vi "log analysis_gps.vi"() -> ()   [LabVIEW 2019] (continued)
system status\tnormal 2 28.000000 0 0\trobot status\t283.924052\t71.154342\t9.753100\t-0.332297\t-2.244729\t149.990746\t0.281000\t0.028000\n\t\n15:33:22.5\tlog_raw\tgps_raw\t#DUALANTENNAHEADINGA,USB3,0,50.5,FINESTEERING,2107,282820.500,02008000,d426,15824;INSUFFICIENT_OBS,NONE,-1.000000000,0.000000000,0.000000000,0.0,0.000000000,0.000000000,\"631T\",14,2,2,2,04,00,20,00*d6a33192\n\tsystem status\tnormal 2 28.000000 0 0\trobot status\t283.808490\t71.236602\t9.749900\t-0.277262\t-2.162787\t150.076452\t0.284000\t0.021000\n\t\n15:33:23.0\tlog_raw\tgps_raw\t#DUALANTENNAHEADINGA,USB3,0,50.5,FINESTEERING,2107,282821.000,02008000,d426,15824;INSUFFICIENT_OBS,NONE,-1.000000000,0.000000000,0.000000000,0.0,0.000000000,0.000000000,\"631T\",16,2,2,2,04,00,20,00*18dc22e3\n\tsystem status\tnormal 2 28.000000 0 0\trobot status\t283.690413\t71.319846\t9.746300\t-0.267508\t-2.122984\t150.127557\t0.314000\t-0.023000\n\t\n15:33:23.5\tlog_raw\tgps_raw\t\tsystem status\tnormal 2 28.000000 0 0\trobot status\t283.569355\t71.402549\t9.742500\t-0.374264\t-1.857958\t150.068560\t0.286000\t0.008000\n\t\n15:33:24.0\tlog_raw\tgps_raw\t#DUALANTENNAHEADINGA,USB3,0,50.0,FINESTEERING,2107,282822.000,02008000,d426,15824;INSUFFICIENT_OBS,NONE,-1.000000000,0.000000000,0.000000000,0.0,0.000000000,0.000000000,\"631T\",16,2,2,2,04,00,20,00*fbcec944\n\tsystem status\tnormal 2 28.000000 0 0\trobot status\t283.449551\t71.484070\t9.737500\t-0.512487\t-1.771439\t150.084314\t0.227000\t0.089000\n\t\n15:33:24.5\tlog_raw\tgps_raw\t#DUALANTENNAHEADINGA,USB3,0,49.0,FINESTEERING,2107,282822.500,02008000,d426,15824;INSUFFICIENT_OBS,NONE,-1.000000000,0.000000000,0.000000000,0.0,0.000000000,0.000000000,\"631T\",15,2,2,2,04,00,20,00*aed41295\n\tsystem status\tnormal 2 28.000000 0 0\trobot status\t283.332205\t71.563886\t9.733200\t-0.549068\t-1.653823\t150.119212\t0.315000\t-0.042000\n\t\n15:33:25.0\tlog_raw\tgps_raw\t#DUALANTENNAHEADINGA,USB3,0,49.0,FINESTEERING,2107,282823.000,02008000,d426,15824;INSUFFICIENT_OBS,NONE,-1.000000000,0.000000000,0.000000000,0.0,0.000000000,0.000000000,\"631T\",15,2,2,2,04,00,20,00*141f0715\n\tsystem status\tnormal 2 28.000000 0 0\trobot status\t283.211432\t71.646224\t9.728200\t-0.568064\t-1.487508\t150.090208\t0.360000\t-0.109000\n\t\n15:33:25.5\tlog_raw\tgps_raw\t#DUALANTENNAHEADINGA,USB3,0,45.5,FINESTEERING,2107,282823.500,02008000,d426,15824;INSUFFICIENT_OBS,NONE,-1.000000000,0.000000000,0.000000000,0.0,0.000000000,0.000000000,\"631T\",14,2,2,2,04,00,20,00*9f3295ab\n\tsystem status\tnormal 2 28.000000 0 0\trobot status\t283.090999\t71.728498\t9.724600\t-0.461891\t-1.625823\t149.976629\t0.307000\t-0.003000\n\t\n15:33:26.0\tlog_raw\tgps_raw\t#DUALANTENNAHEADINGA,USB3,0,45.5,FINESTEERING,2107,282824.000,02008000,d426,15824;INSUFFICIENT_OBS,NONE,-1.000000000,0.000000000,0.000000000,0.0,0.000000000,0.000000000,\"631T\",12,2,2,2,04,00,20,00*0f8497af\n\tsystem status\tnormal 2 28.000000 0 0\trobot status\t282.974020\t71.807251\t9.720400\t-0.558474\t-1.792565\t149.954982\t0.295000\t0.003000\n\t\n15:33:26.5\tlog_raw\tgps_raw\t#DUALANTENNAHEADINGA,USB3,0,50.5,FINESTEERING,2107,282824.500,02000000,d426,15824;INSUFFICIENT_OBS,NONE,-1.000000000,0.000000000,0.000000000,0.0,0.000000000,0.000000000,\"631T\",12,2,2,2,04,00,20,00*31fdab05\n\tsystem status\tnormal 2 28.000000 0 0\trobot status\t282.850810\t71.889210\t9.716700\t-0.699481\t-2.078597\t149.902824\t0.242000\t0.068000\n\t\n15:33:27.0\tlog_raw\tgps_raw\t#DUALANTENNAHEADINGA,USB3,0,50.5,FINESTEERING,2107,282825.000,02000000,d426,15824;INSUFFICIENT_OBS,NONE,-1.000000000,0.000000000,0.000000000,0.0,0.000000000,0.000000000,\"631T\",14,2,2,2,04,00,20,00*16eab596\n\tsystem status\tnormal 2 28.000000 0 0\trobot status\t282.725956\t71.973215\t9.713500\t-0.651887\t-2.450646\t149.804912\t0.365000\t-0.098000\n\t\n15:33:27.5\tlog_raw\tgps_raw\t#DUALANTENNAHEADINGA,USB3,0,49.5,FINESTEERING,2107,282825.500,02000000,d426,15824;INSUFFICIENT_OBS,NONE,-1.000000000,0.000000000,0.000000000,0.0,0.000000000,0.000000000,\"631T\",16,2,2,2,04,00,20,00*9412ee1f\n\tsystem status\tnormal 2 28.000000 0 0\trobot status\t282.610464\t72.054506\t9.710700\t-0.484140\t-2.602486\t149.755855\t0.326000\t-0.026000\n\t\n15:33:28.0\tlog_raw\tgps_raw\t#DUALANTENNAHEADINGA,USB3,0,49.5,FINESTEERING,2107,282826.000,02000000,d426,15824;INSUFFICIENT_OBS,NONE,-1.000000000,0.000000000,0.000000000,0.0,0.000000000,0.000000000,\"631T\",15,2,2,2,04,00,20,00*563f7484\n\tsystem status\tnormal 2 28.000000 0 0\trobot status\t282.494849\t72.134469\t9.707100\t-0.504429\t-2.557112\t149.697525\t0.254000\t0.039000\n\t\n15:33:28.5\tlog_raw\tgps_raw\t\tsystem status\tnormal 2 28.000000 0 0\trobot status\t282.373086\t72.218767\t9.703200\t-0.635839\t-2.212049\t149.570497\t0.320000\t-0.037000\n\t\n15:33:29.0\tlog_raw\tgps_raw\t#DUALANTENNAHEADINGA,USB3,0,48.5,FINESTEERING,2107,282827.000,02000000,d426,15824;INSUFFICIENT_OBS,NONE,-1.000000000,0.000000000,0.000000000,0.0,0.000000000,0.000000000,\"631T\",15,2,2,2,04,00,20,00*5fa3a6f9\n\tsystem status\tnormal 2 28.000000 0 0\trobot status\t282.257571\t72.299769\t9.697900\t-0.652077\t-1.944229\t149.541752\t0.281000\t0.018000\n\t\n15:33:29.5\tlog_raw\tgps_raw\t#DUALANTENNAHEADINGA,USB3,0,47.0,FINESTEERING,2107,282827.500,02000000,d426,15824;INSUFFICIENT_OBS,NONE,-1.000000000,0.000000000,0.000000000,0.0,0.000000000,0.000000000,\"631T\",14,2,2,2,04,00,20,00*78434fab\n\tsystem status\tnormal 2 28.000000 0 0\trobot status\t282.145140\t72.380480\t9.693600\t-0.557379\t-1.847742\t149.470540\t0.314000\t-0.010000\n\t\n15:33:30.0\tlog_raw\tgps_raw\t#DUALANTENNAHEADINGA,USB3,0,47.0,FINESTEERING,2107,282828.000,02000000,d426,15824;INSUFFICIENT_OBS,NONE,-1.000000000,0.000000000,0.000000000,0.0,0.000000000,0.000000000,\"631T\",14,2,2,2,04,00,20,00*ad0b6cf6\n\tsystem status\tnormal 2 28.000000 0 0\trobot status\t282.021945\t72.467157\t9.688800\t-0.594870\t-1.866738\t149.388491\t0.256000\t0.059000\n\t\n15:33:30.5\tlog_raw\tgps_raw\t#DUALANTENNAHEADINGA,USB3,0,50.0,FINESTEERING,2107,282828.500,02000000,d426,15824;INSUFFICIENT_OBS,NONE,-1.000000000,0.000000000,0.000000000,0.0,0.000000000,0.000000000,\"631T\",14,2,2,2,04,00,20,00*4d6879b5\n\tsystem status\tnormal 2 28.000000 0 0\trobot status\t281.914611\t72.542750\t9.686000\t-0.692895\t-1.958768\t149.311911\t0.298000\t-0.008000\n\t\n15:33:31.0\tlog_raw\tgps_raw\t#DUALANTENNAHEADINGA,USB3,0,50.0,FINESTEERING,2107,282829.000,02000000,d426,15824;INSUFFICIENT_OBS,NONE,-1.000000000,0.000000000,0.000000000,0.0,0.000000000,0.000000000,\"631T\",14,2,2,2,04,00,20,00*f7a36c35\n\tsystem status\tnormal 2 28.000000 0 0\trobot status\t281.794350\t72.627065\t9.683000\t-0.746278\t-2.115926\t149.154539\t0.312000\t-0.014000\n\t\n15:33:31.5\tlog_raw\tgps_raw\t#DUALANTENNAHEADINGA,USB3,0,51.0,FINESTEERING,2107,282829.500,02000000,d426,15824;INSUFFICIENT_OBS,NONE,-1.000000000,0.000000000,0.000000000,0.0,0.000000000,0.000000000,\"631T\",15,2,2,2,04,00,20,00*93162b90\n\tsystem status\tnormal 2 28.000000 0 0\trobot status\t281.681853\t72.708661\t9.679700\t-0.908283\t-2.116420\t149.030065\t0.293000\t0.000000\n\t\n15:33:32.0\tlog_raw\tgps_raw\t#INSPVAXA,USB3,0,51.0,FINESTEERING,2107,282830.050,02000000,471d,15824;INS_ALIGNMENT_COMPLETE,INS_RTKFIXED,37.37078622103,126.72401367008,9.6748,22.3000,0.1678,-0.2481,-0.0115,-0.997229556,-1.986004946,301.087266314,0.4437,0.2943,0.5539,0.1140,0.0924,0.0773,0.0983,0.1033,4.8231,0f000001,0*4fbfc59a\n\tsystem status\tnormal 2 28.000000 0 0\trobot status\t281.552080\t72.803878\t9.674800\t-0.997230\t-1.986005\t148.912734\t0.303000\t-0.014000\n\t\n15:33:32.5\tlog_raw\tgps_raw\t\tsystem status\tnormal 2 28.000000 0 0\trobot status\t281.447458\t72.881989\t9.670700\t-0.873866\t-2.088030\t148.867569\t0.243000\t0.080000\n\t\n15:33:33.0\tlog_raw\tgps_raw\t#DUALANTENNAHEADINGA,USB3,0,51.5,FINESTEERING,2107,282831.000,02000000,d426,15824;INSUFFICIENT_OBS,NONE,-1.000000000,0.000000000,0.000000000,0.0,0.000000000,0.000000000,\"631T\",14,2,2,2,04,00,20,00*e1ddc463\n\tsystem status\tnormal 2 28.000000 0 0\trobot status\t281.344907\t72.958986\t9.667500\t-0.891921\t-2.101473\t148.771989\t0.306000\t0.004000\n\t\n15:33:33.5\tlog_raw\tgps_raw\t#INSPVAXA,USB3,0,50.0,FINESTEERING,2107,282831.550,02000000,471d,15824;INS_ALIGNMENT_COMPLETE,INS_RTKFIXED,37.37078850340,126.72400981553,9.6631,22.3000,0.1496,-0.2201,-0.0118,-1.048727398,-2.216278260,301.282066784,0.4433,0.2942,0.5538,0.1139,0.0924,0.0773,0.0983,0.1033,4.8246,0f000001,0*7f01e368\n\tsystem status\tnormal 2 28.000000 0 0\trobot status\t281.210650\t73.057197\t9.663100\t-1.048727\t-2.216278\t148.717933\t0.357000\t-0.084000\n\t\n15:33:34.0\tlog_raw\tgps_raw\t\tsystem status\tnormal 2 28.000000 0 0\trobot status\t281.116346\t73.129707\t9.659100\t-0.942578\t-2.240698\t148.610781\t0.298000\t-0.003000\n\t\n15:33:34.5\tlog_raw\tgps_raw\t#DUALANTENNAHEADINGA,USB3,0,47.0,FINESTEERING,2107,282832.500,02000000,d426,15824;INSUFFICIENT_OBS,NONE,-1.000000000,0.000000000,0.000000000,0.0,0.000000000,0.000000000,\"631T\",16,2,2,2,04,00,20,00*f25cead2\n\tsystem status\tnormal 2 28.000000 0 0\trobot status\t280.998531\t73.218930\t9.655300\t-0.833231\t-2.237985\t148.504375\t0.276000\t0.029000\n\t\n15:33:35.0\tlog_raw\tgps_raw\t#INSPVAXA,USB3,0,47.0,FINESTEERING,2107,282833.050,02000000,471d,15824;INS_ALIGNMENT_COMPLETE,INS_RTKFIXED,37.37079076592,126.72400610442,9.6518,22.3000,0.1650,-0.2502,-0.0160,-0.860770994,-2.117713519,301.563204490,0.4421,0.2941,0.5532,0.1138,0.0924,0.0773,0.0983,0.1033,4.8276,0f000001,0*c29dada0\n\tsystem status\tnormal 2 28.000000 0 0\trobot status\t280.881926\t73.308313\t9.651800\t-0.860771\t-2.117714\t148.436796\t0.306000\t0.000000\n\t\n15:33:35.5\tlog_raw\tgps_raw\t#DUALANTENNAHEADINGA,USB3,0,50.5,FINESTEERING,2107,282833.500,02000000,d426,15824;INSUFFICIENT_OBS,NONE,-1.000000000,0.000000000,0.000000000,0.0,0.000000000,0.000000000,\"631T\",14,2,2,2,04,00,20,00*893a0a2c\n\tsystem status\tnormal 2 28.000000 0 0\trobot status\t280.776396\t73.388077\t9.648000\t-0.874609\t-2.150873\t148.396539\t0.288000\t0.021000\n\t\n15:33:36.0\tlog_raw\tgps_raw\t\tsystem status\tnormal 2 28.000000 0 0\trobot status\t280.665453\t73.473365\t9.643900\t-0.840149\t-2.187439\t148.407207\t0.311000\t-0.011000\n\t\n15:33:36.5\tlog_raw\tgps_raw\t#DUALANTENNAHEADINGA,USB3,0,47.5,FINESTEERING,2107,282834.500,02000000,d426,15824;INSUFFICIENT_OBS,NONE,-1.000000000,0.000000000,0.000000000,0.0,0.000000000,0.000000000,\"631T\",16,2,2,2,04,00,20,00*10871089\n\tsystem status\tnormal 2 28.000000 0 0\trobot status\t280.559684\t73.555042\t9.640800\t-0.892122\t-2.049561\t148.485363\t0.264000\t0.084000\n\t\n15:33:37.0\tlog_raw\tgps_raw\t#INSPVAXA,USB3,0,47.5,FINESTEERING,2107,282835.050,02000000,471d,15824;INS_ALIGNMENT_COMPLETE,INS_RTKFIXED,37.37079382962,126.72400108801,9.6374,22.3000,0.1569,-0.2281,-0.0111,-0.999674572,-2.085636983,301.443482379,0.4416,0.2941,0.5526,0.1138,0.0924,0.0773,0.0983,0.1033,4.8306,0f000001,0*021b0f77\n\tsystem status\tnormal 2 27.900000 0 0\trobot status\t280.437581\t73.648351\t9.637400\t-0.999675\t-2.085637\t148.556518\t0.292000\t0.012000\n\t\n15:33:37.5\tlog_raw\tgps_raw\t#INSPVAXA,USB3,0,49.0,FINESTEERING,2107,282835.550,02000000,471d,15824;INS_ALIGNMENT_COMPLETE,INS_RTKFIXED,37.37079461184,126.72399982045,9.6347,22.3000,0.1482,-0.2050,-0.0185,-0.996168603,-2.046587812,301.390130143,0.4416,0.2941,0.5526,0.1138,0.0924,0.0773,0.0983,0.1033,4.8306,0f000001,0*e466e7db\n\tsystem status\tnormal 2 28.000000 0 0\trobot status\t280.325302\t73.735169\t9.634700\t-0.996169\t-2.046588\t148.609870\t0.244000\t0.080000\n\t\n15:33:38.0\tlog_raw\tgps_raw\t\tsystem status\tnormal 2 28.000000 0 0\trobot status\t280.227304\t73.813414\t9.632200\t-0.822483\t-2.094044\t148.714421\t0.376000\t-0.124000\n\t\n15:33:38.5\tlog_raw\tgps_raw\t#INSPVAXA,USB3,0,49.5,FINESTEERING,2107,282836.550,02000000,471d,15824;INS_ALIGNMENT_COMPLETE,INS_RTKFIXED,37.37079614762,126.72399733501,9.6280,22.3000,0.1600,-0.2167,-0.0303,-0.871497210,-2.188105469,301.034385182,0.4418,0.2941,0.5524,0.1139,0.0924,0.0773,0.0983,0.1033,4.8319,0f000001,0*58ef0c84\n\tsystem status\tnormal 2 27.900000 0 0\trobot status\t280.105146\t73.905625\t9.628000\t-0.871497\t-2.188105\t148.965615\t0.289000\t0.036000\n\t\n15:33:39.0\tlog_raw\tgps_raw\t#INSPVAXA,USB3,0,48.5,FINESTEERING,2107,282837.050,02000000,471d,15824;INS_ALIGNMENT_COMPLETE,INS_RTKFIXED,37.37079689035,126.72399612134,9.6249,22.3000,0.1550,-0.2065,-0.0179,-0.785589438,-2.162266254,300.814007904,0.4425,0.2941,0.5525,0.1140,0.0924,0.0773,0.0983,0.1033,4.8330,0f000001,0*63c71cff\n\tsystem status\tnormal 2 28.000000 0 0\trobot status\t279.997641\t73.988060\t9.624900\t-0.785589\t-2.162266\t149.185992\t0.330000\t-0.034000\n\t\n15:33:39.5\tlog_raw\tgps_raw\t#INSPVAXA,USB3,0,48.5,FINESTEERING,2107,282837.550,02000000,471d,15824;INS_ALIGNMENT_COMPLETE,INS_RTKFIXED,37.37079762799,126.72399488402,9.6202,22.3000,0.1524,-0.1993,-0.0171,-0.713862007,-2.052581994,300.562898535,0.4425,0.2941,0.5525,0.1140,0.0924,0.0773,0.0983,0.1033,4.8330,0f000001,0*d3644a20\n\tsystem status\tnormal 2 27.900000 0 0\trobot status\t279.888041\t74.069930\t9.620200\t-0.713862\t-2.052582\t149.437101\t0.275000\t0.040000\n\t\n15:33:40.0\tlog_raw\tgps_raw\t\tsystem status\tnormal 2 27.900000 0 0\trobot status\t279.790123\t74.141776\t9.616300\t-0.772465\t-1.876222\t149.672346\t0.287000\t0.025000\n\t\n15:33:40.5\tlog_raw\tgps_raw\t#INSPVAXA,USB3,0,49.5,FINESTEERING,2107,282838.550,02000000,471d,15824;INS_ALIGNMENT_COMPLETE,INS_RTKFIXED,37.37079907064,126.72399237464,9.6125,22.3000,0.1577,-0.2192,-0.0140,-0.837165227,-1.670419356,300.018600301,0.4429,0.2941,0.5524,0.1143,0.0924,0.0773,0.0982,0.1033,4.8338,0f000001,0*758de772\n\tsystem status\tnormal 2 27.900000 0 0\trobot status\t279.665765\t74.230050\t9.612500\t-0.837165\t-1.670419\t149.981400\t0.281000\t0.051000\n\t\n15:33:41.0\tlog_raw\tgps_raw\t#INSPVAXA,USB3,0,49.5,FINESTEERING,2107,282839.050,02000000,471d,15824;INS_ALIGNMENT_COMPLETE,INS_RTKFIXED,37.37079978171,126.72399113225,9.6082,22.3000,0.1499,-0.2017,-0.0243,-0.847366438,-1.584995837,299.787057757,0.4435,0.2941,0.5523,0.1144,0.0925,0.0773,0.0982,0.1033,4.8337,0f000001,0*2af0ce7f\n\tsystem status\tnormal 2 28.000000 0 0\trobot status\t279.555716\t74.308971\t9.608200\t-0.847366\t-1.584996\t150.212942\t0.232000\t0.102000\n\t\n15:33:41.5\tlog_raw\tgps_raw\t#INSPVAXA,USB3,0,51.0,FINESTEERING,2107,282839.550,02000000,471d,15824;INS_ALIGNMENT_COMPLETE,INS_RTKFIXED,37.37080052394,126.72398985335,9.6041,22.3000,0.1541,-0.2085,-0.0197,-0.657538582,-1.555388056,299.628697476,0.4435,0.2941,0.5523,0.1144,0.0925,0.0773,0.0982,0.1033,4.8337,0f000001,0*e249b229\n\tsystem status\tnormal 2 27.900000 0 0\trobot status\t279.442433\t74.391351\t9.604100\t-0.657539\t-1.555388\t150.371303\t0.344000\t-0.076000\n\t\n15:33:42.0\tlog_raw\tgps_raw\t\tsystem status\tnormal 2 27.900000 0 0\trobot status\t279.341493\t74.463887\t9.599600\t-0.599535\t-1.617170\t150.501142\t0.347000\t-0.060000\n\t\n15:33:42.5\tlog_raw\tgps_raw\t#INSPVAXA,USB3,0,50.5,FINESTEERING,2107,282840.550,02000000,471d,15824;INS_ALIGNMENT_COMPLETE,INS_RTKFIXED,37.37080198086,126.72398726607,9.5945,22.3000,0.1415,-0.2075,-0.0192,-0.681588994,-1.930393004,299.482671572,0.4442,0.2942,0.5523,0.1142,0.0924,0.0773,0.0982,0.1033,4.8325,0f000001,0*f7245bcc\n\tsystem status\tnormal 2 28.000000 0 0\trobot status\t279.213256\t74.553054\t9.594500\t-0.681589\t-1.930393\t150.517328\t0.275000\t0.043000\n\t\n15:33:43.0\tlog_raw\tgps_raw\t#INSPVAXA,USB3,0,50.5,FINESTEERING,2107,282841.050,02000000,471d,15824;INS_ALIGNMENT_COMPLETE,INS_RTKFIXED,37.37080269801,126.72398599204,9.5896,22.3000,0.1407,-0.1883,-0.0149,-0.746862353,-2.032009103,299.450305657,0.4442,0.2942,0.5522,0.1141,0.0924,0.0773,0.0982,0.1032,4.8310,0f000001,0*0739b113\n\tsystem status\tnormal 2 27.900000 0 0\trobot status\t279.100404\t74.632651\t9.589600\t-0.746862\t-2.032009\t150.549694\t0.243000\t0.088000\n\t\n15:33:43.5\tlog_raw\tgps_raw\t#INSPVAXA,USB3,0,47.0,FINESTEERING,2107,282841.550,02000000,471d,15824;INS_ALIGNMENT_COMPLETE,INS_RTKFIXED,37.37080343630,126.72398465654,9.5859,22.3000,0.1441,-0.2016,-0.0158,-0.831480071,-2.195246795,299.385489807,0.4442,0.2942,0.5522,0.1141,0.0924,0.0773,0.0982,0.1032,4.8310,0f000001,0*a0ec8594\n\tsystem status\tnormal 2 28.000000 0 0\trobot status\t278.982108\t74.714594\t9.585900\t-0.831480\t-2.195247\t150.614510\t0.197000\t0.147000\n\t\n15:33:44.0\tlog_raw\tgps_raw\t#INSPVAXA,USB3,0,46.5,FINESTEERING,2107,282842.050,02000000,471d,15824;INS_ALIGNMENT_COMPLETE,INS_RTKFIXED,37.37080417345,126.72398334114,9.5820,22.3000,0.1511,-0.2042,-0.0206,-0.794633403,-2.254519225,299.313785412,0.4438,0.2942,0.5520,0.1137,0.0924,0.0772,0.0982,0.1032,4.8295,0f000001,0*390828f0\n\tsystem status\tnormal 2 28.000000 0 0\trobot status\t278.865592\t74.796410\t9.582000\t-0.794633\t-2.254519\t150.686215\t0.359000\t-0.079000\n\t\n15:33:44.5\tlog_raw\tgps_raw\t#INSPVAXA,USB3,0,46.5,FINESTEERING,2107,282842.550,02000000,471d,15824;INS_ALIGNMENT_COMPLETE,INS_RTKFIXED,37.37080492291,126.72398204575,9.5781,22.3000,0.1466,-0.2045,-0.0217,-0.587846537,-2.261082521,299.368921912,0.4438,0.2942,0.5520,0.1137,0.0924,0.0772,0.0982,0.1032,4.8295,0f000001,0*9ddbd7c7\n\tsystem status\tnormal 2 28.000000 0 0\trobot status\t278.750848\t74.879592\t9.578100\t-0.587847\t-2.261083\t150.631078\t0.370000\t-0.112000\n\t\n15:33:45.0\tlog_raw\tgps_raw\t#INSPVAXA,USB3,0,46.5,FINESTEERING,2107,282843.050,02000000,471d,15824;INS_ALIGNMENT_COMPLETE,INS_RTKFIXED,37.37080566870,126.72398074821,9.5741,22.3000,0.1339,-0.1915,-0.0133,-0.480026925,-2.203118399,299.401112268,0.4434,0.2940,0.5520,0.1139,0.0924,0.0772,0.0981,0.1031,4.8288,0f000001,0*1d5f5b91\n\tsystem status\tnormal 2 28.000000 0 0\trobot status\t278.635914\t74.962367\t9.574100\t-0.480027\t-2.203118\t150.598888\t0.232000\t0.073000\n\t\n15:33:45.5\tlog_raw\tgps_raw\t#INSPVAXA,USB3,0,48.0,FINESTEERING,2107,282843.550,02000000,471d,15824;INS_ALIGNMENT_COMPLETE,INS_RTKFIXED,37.37080641021,126.72397942469,9.5707,22.3000,0.1423,-0.2057,-0.0134,-0.517073533,-2.121653000,299.405019145,0.4434,0.2940,0.5520,0.1139,0.0924,0.0772,0.0981,0.1031,4.8288,0f000001,0*aad3db2c\n\tsystem status\tnormal 2 28.000000 0 0\trobot status\t278.518679\t75.044667\t9.570700\t-0.517074\t-2.121653\t150.594981\t0.294000\t0.003000\n\t\n15:33:46.0\tlog_raw\tgps_raw\t\tsystem status\tnormal 2 28.000000 0 0\trobot status\t278.416737\t75.118075\t9.567400\t-0.558894\t-2.003107\t150.535658\t0.290000\t0.009000\n\t\n15:33:46.5\tlog_raw\tgps_raw\t#DUALANTENNAHEADINGA,USB3,0,46.5,FINESTEERING,2107,282844.500,02000000,d426,15824;INSUFFICIENT_OBS,NONE,-1.000000000,0.000000000,0.000000000,0.0,0.000000000,0.000000000,\"631T\",14,2,2,2,04,00,20,00*91c9d553\n\tsystem status\tnormal 2 28.000000 0 0\trobot status\t278.297706\t75.202632\t9.562500\t-0.471081\t-2.062458\t150.489849\t0.272000\t0.017000\n\t\n15:33:47.0\tlog_raw\tgps_raw\t#INSPVAXA,USB3,0,46.5,FINESTEERING,2107,282845.050,02000000,471d,15824;INS_ALIGNMENT_COMPLETE,INS_RTKFIXED,37.37080866547,126.72397546111,9.5573,22.3000,0.1531,-0.2061,-0.0195,-0.434360785,-2.083992757,299.534678946,0.4435,0.2939,0.5519,0.1137,0.0924,0.0772,0.0981,0.1031,4.8277,0f000001,0*84ceebbb\n\tsystem status\tnormal 2 28.000000 0 0\trobot status\t278.167592\t75.294978\t9.557300\t-0.434361\t-2.083993\t150.465321\t0.247000\t0.077000\n\t\n15:33:47.5\tlog_raw\tgps_raw\t#INSPVAXA,USB3,0,48.5,FINESTEERING,2107,282845.550,02000000,471d,15824;INS_ALIGNMENT_COMPLETE,INS_RTKFIXED,37.37080941702,126.72397412031,9.5548,22.3000,0.1626,-0.2203,-0.0192,-0.594420667,-2.098021967,299.551674256,0.4435,0.2939,0.5519,0.1137,0.0924,0.0772,0.0981,0.1031,4.8277,0f000001,0*c2a985dc\n\tsystem status\tnormal 2 28.000000 0 0\trobot status\t278.048826\t75.378393\t9.554800\t-0.594421\t-2.098022\t150.448326\t0.371000\t-0.099000\n\t\n15:33:48.0\tlog_raw\tgps_raw\t#INSPVAXA,USB3,0,47.5,FINESTEERING,2107,282846.050,02000000,471d,15824;INS_ALIGNMENT_COMPLETE,INS_RTKFIXED,37.37081017945,126.72397278683,9.5521,22.3000,0.1549,-0.2109,-0.0140,-0.604914668,-2.152808656,299.610978470,0.4432,0.2939,0.5518,0.1137,0.0924,0.0772,0.0981,0.1031,4.8275,0f000001,0*a6608b47\n\tsystem status\tnormal 2 28.000000 0 0\trobot status\t277.930708\t75.463014\t9.552100\t-0.604915\t-2.152809\t150.389022\t0.259000\t0.059000\n\t\n15:33:48.5\tlog_raw\tgps_raw\t#INSPVAXA,USB3,0,47.5,FINESTEERING,2107,282846.550,02000000,471d,15824;INS_ALIGNMENT_COMPLETE,INS_RTKFIXED,37.37081095004,126.72397139929,9.5473,22.3000,0.1385,-0.1894,-0.0029,-0.694805946,-2.128009753,299.688157025,0.4432,0.2939,0.5518,0.1137,0.0924,0.0772,0.0981,0.1031,4.8275,0f000001,0*5d110ef8\n\tsystem status\tnormal 2 28.000000 0 0\trobot status\t277.807802\t75.548542\t9.547300\t-0.694806\t-2.128010\t150.311843\t0.248000\t0.063000\n\t\n15:33:49.0\tlog_raw\tgps_raw\t#INSPVAXA,USB3,0,44.5,FINESTEERING,2107,282847.050,02000000,471d,15824;INS_ALIGNMENT_COMPLETE,INS_RTKFIXED,37.37081171742,126.72397003068,9.5427,22.3000,0.1573,-0.2192,-0.0020,-0.777578191,-2.007727791,299.761533607,0.4435,0.2940,0.5521,0.1137,0.0924,0.0772,0.0981,0.1031,4.8277,0f000001,0*78548d8e\n\tsystem status\tnormal 2 28.000000 0 0\trobot status\t277.686573\t75.633714\t9.542700\t-0.777578\t-2.007728\t150.238466\t0.313000\t-0.016000\n\t\n15:33:49.5\tlog_raw\tgps_raw\t#INSPVAXA,USB3,0,44.5,FINESTEERING,2107,282847.550,02000000,471d,15824;INS_ALIGNMENT_COMPLETE,INS_RTKFIXED,37.37081244961,126.72396875131,9.5405,22.3000,0.1641,-0.2218,-0.0106,-0.802151330,-1.920952187,299.784241204,0.4435,0.2940,0.5521,0.1137,0.0924,0.0772,0.0981,0.1031,4.8277,0f000001,0*07f3c654\n\tsystem status\tnormal 2 28.000000 0 0\trobot status\t277.573249\t75.714979\t9.540500\t-0.802151\t-1.920952\t150.215759\t0.314000\t-0.006000\n\t\n15:33:50.0\tlog_raw\tgps_raw\t#INSPVAXA,USB3,0,44.5,FINESTEERING,2107,282848.050,02000000,471d,15824;INS_ALIGNMENT_COMPLETE,INS_RTKFIXED,37.37081323454,126.72396738661,9.5387,22.3000,0.1349,-0.1756,0.0025,-0.775318763,-1.846543645,299.874004513,0.4431,0.2940,0.5522,0.1139,0.0924,0.0772,0.0981,0.1031,4.8282,0f000001,0*cf4a726c\n\tsystem status\tnormal 2 28.000000 0 0\trobot status\t277.452366\t75.802098\t9.538700\t-0.775319\t-1.846544\t150.125995\t0.270000\t0.029000\n\t\n15:33:50.5\tlog_raw\tgps_raw\t#INSPVAXA,USB3,0,45.0,FINESTEERING,2107,282848.550,02000000,471d,15824;INS_ALIGNMENT_COMPLETE,INS_RTKFIXED,37.37081402726,126.72396600462,9.5360,22.3000,0.1572,-0.2154,0.0012,-0.746342979,-1.873663068,299.943587251,0.4431,0.2940,0.5522,0.1139,0.0924,0.0772,0.0981,0.1031,4.8282,0f000001,0*b8902195\n\tsystem status\tnormal 2 28.000000 0 0\trobot status\t277.329951\t75.890082\t9.536000\t-0.746343\t-1.873663\t150.056413\t0.362000\t-0.094000\n\t\n15:33:51.0\tlog_raw\tgps_raw\t#INSPVAXA,USB3,0,44.5,FINESTEERING,2107,282849.050,02000000,471d,15824;INS_ALIGNMENT_COMPLETE,INS_RTKFIXED,37.37081477161,126.72396469278,9.5343,22.3000,0.1752,-0.2340,-0.0030,-0.967406994,-1.848268930,299.977215039,0.4433,0.2941,0.5523,0.1136,0.0924,0.0772,0.0981,0.1031,4.8286,0f000001,0*2493a191\n\tsystem status\tnormal 2 28.000000 0 0\trobot status\t277.213751\t75.972697\t9.534300\t-0.967407\t-1.848269\t150.022785\t0.302000\t0.019000\n\t\n15:33:51.5\tlog_raw\tgps_raw\t#INSPVAXA,USB3,0,44.5,FINESTEERING,2107,282849.550,02000000,471d,15824;INS_ALIGNMENT_COMPLETE,INS_RTKFIXED,37.37081552203,126.72396337229,9.5340,22.3000,0.1625,-0.2097,0.0040,-0.944405978,-1.796098220,300.013826004,0.4433,0.2941,0.5523,0.1136,0.0924,0.0772,0.0981,0.1031,4.8286,0f000001,0*6a619609\n\tsystem status\tnormal 2 28.000000 0 0\trobot status\t277.096784\t76.055986\t9.534000\t-0.944406\t-1.796098\t149.986174\t0.283000\t0.023000\n\t\n15:33:52.0\tlog_raw\tgps_raw\t#INSPVAXA,USB3,0,44.5,FINESTEERING,2107,282850.050,02000000,471d,15824;INS_ALIGNMENT_COMPLETE,INS_RTKFIXED,37.37081628430,126.72396202369,9.5336,22.3000,0.1377,-0.1761,0.0033,-0.977356975,-1.557691035,300.050326514,0.4426,0.2941,0.5523,0.1138,0.0925,0.0772,0.0981,0.1030,4.8295,0f000001,0*a61f27a1\n\tsystem status\tnormal 2 28.000000 0 0\trobot status\t276.977327\t76.140590\t9.533600\t-0.977357\t-1.557691\t149.949673\t0.343000\t-0.082000\n\t\n15:33:52.5\tlog_raw\tgps_raw\t#INSPVAXA,USB3,0,47.5,FINESTEERING,2107,282850.550,02000000,471d,15824;INS_ALIGNMENT_COMPLETE,INS_RTKFIXED,37.37081707791,126.72396063586,9.5326,22.3000,0.1576,-0.1997,0.0014,-0.911286398,-1.407612709,300.113222709,0.4426,0.2941,0.5523,0.1138,0.0925,0.0772,0.0981,0.1030,4.8295,0f000001,0*c59ed98f\n\tsystem status\tnormal 2 28.000000 0 0\trobot status\t276.854395\t76.228673\t9.532600\t-0.911286\t-1.407613\t149.886777\t0.255000\t0.069000\n\t\n15:33:53.0\tlog_raw\tgps_raw\t#INSPVAXA,USB3,0,47.5,FINESTEERING,2107,282851.050,02000000,471d,15824;INS_ALIGNMENT_COMPLETE,INS_RTKFIXED,37.37081784915,126.72395932045,9.5307,22.3000,0.1604,-0.2227,0.0007,-0.811075284,-1.430938970,300.158787074,0.4420,0.2942,0.5520,0.1135,0.0924,0.0772,0.0981,0.1030,4.8299,0f000001,0*3724944b\n\tsystem status\tnormal 2 28.000000 0 0\trobot status\t276.737879\t76.314273\t9.530700\t-0.811075\t-1.430939\t149.841213\t0.256000\t0.068000\n\t\n15:33:53.5\tlog_raw\tgps_raw\t#INSPVAXA,USB3,0,50.0,FINESTEERING,2107,282851.550,02000000,471d,15824;INS_ALIGNMENT_COMPLETE,INS_RTKFIXED,37.37081861345,126.72395800267,9.5292,22.3000,0.1561,-0.2014,0.0080,-0.732820805,-1.409359332,300.160206583,0.4420,0.2942,0.5520,0.1135,0.0924,0.0772,0.0981,0.1030,4.8299,0f000001,0*b9091ec1\n\tsystem status\tnormal 2 28.000000 0 0\trobot status\t276.621152\t76.399102\t9.529200\t-0.732821\t-1.409359\t149.839793\t0.289000\t0.003000\n\t\n15:33:54.0\tlog_raw\tgps_raw\t#INSPVAXA,USB3,0,41.5,FINESTEERING,2107,282852.050,02000000,471d,15824;INS_ALIGNMENT_COMPLETE,INS_RTKFIXED,37.37081939468,126.72395663812,9.5281,22.3000,0.1575,-0.2070,-0.0013,-0.818147595,-1.685386594,300.178906783,0.4415,0.2941,0.5518,0.1134,0.0924,0.0772,0.0981,0.1030,4.8305,0f000001,0*5aa17ff6\n\tsystem status\tnormal 2 28.000000 0 0\trobot status\t276.500282\t76.485811\t9.528100\t-0.818148\t-1.685387\t149.821093\t0.247000\t0.069000\n\t\n15:33:54.5\tlog_raw\tgps_raw\t\tsystem status\tnormal 2 28.000000 0 0\trobot status\t276.379670\t76.570270\t9.525800\t-1.033852\t-1.931821\t149.792185\t0.298000\t0.018000\n\t\n15:33:55.0\tlog_raw\tgps_raw\t\tsystem status\tnormal 2 28.000000 0 0\trobot status\t276.262208\t76.654965\t9.521300\t-1.001174\t-2.073321\t149.795836\t0.264000\t0.068000\n\t\n15:33:55.5\tlog_raw\tgps_raw\t\tsystem status\tnormal 2 27.900000 0 0\trobot status\t276.145482\t76.741148\t9.518200\t-0.826197\t-2.169054\t149.798993\t0.296000\t0.000000\n\t\n15:33:56.0\tlog_raw\tgps_raw\t\tsystem status\tnormal 2 28.000000 0 0\trobot status\t276.026826\t76.827664\t9.515100\t-0.869102\t-2.262425\t149.792215\t0.289000\t0.024000\n\t\n15:33:56.5\tlog_raw\tgps_raw\t\tsystem status\tnormal 2 28.000000 0 0\trobot status\t275.911435\t76.912012\t9.512300\t-0.865437\t-2.274483\t149.779580\t0.286000\t0.026000\n\t\n15:33:57.0\tlog_raw\tgps_raw\t#INSPVAXA,USB3,0,47.5,FINESTEERING,2107,282855.050,02000000,471d,15824;INS_ALIGNMENT_COMPLETE,INS_RTKFIXED,37.37082400176,126.72394869235,9.5093,22.3000,0.1580,-0.2046,-0.0114,-0.756987003,-2.231320148,300.245266772,0.4400,0.2940,0.5516,0.1134,0.0924,0.0772,0.0981,0.1030,4.8343,0f000001,0*a1d38784\n\tsystem status\tnormal 2 28.000000 0 0\trobot status\t275.796459\t76.997149\t9.509300\t-0.756987\t-2.231320\t149.754733\t0.243000\t0.086000\n\t\n15:33:57.5\tlog_raw\tgps_raw\t#INSPVAXA,USB3,0,48.0,FINESTEERING,2107,282855.550,02000000,471d,15824;INS_ALIGNMENT_COMPLETE,INS_RTKFIXED,37.37082475865,126.72394738015,9.5053,22.3000,0.1620,-0.1986,-0.0100,-0.702343381,-2.122687121,300.199626754,0.4400,0.2940,0.5516,0.1134,0.0924,0.0772,0.0981,0.1030,4.8343,0f000001,0*af41ec57\n\tsystem status\tnormal 2 28.000000 0 0\trobot status\t275.680226\t77.081156\t9.505300\t-0.702343\t-2.122687\t149.800373\t0.372000\t-0.123000\n\t\n15:33:58.0\tlog_raw\tgps_raw\t#INSPVAXA,USB3,0,46.5,FINESTEERING,2107,282856.050,02008000,471d,15824;INS_ALIGNMENT_COMPLETE,INS_RTKFIXED,37.37082551882,126.72394606788,9.5018,22.3000,0.1724,-0.2105,-0.0168,-0.698987302,-1.986256005,300.182498357,0.4393,0.2939,0.5514,0.1133,0.0924,0.0772,0.0981,0.1030,4.8357,0f000001,0*2de35edc\n\tsystem status\tnormal 2 28.000000 0 0\trobot status\t275.563988\t77.165527\t9.501800\t-0.698987\t-1.986256\t149.817502\t0.264000\t0.053000\n\t\n15:33:58.5\tlog_raw\tgps_raw\t\tsystem status\tnormal 2 28.000000 0 0\trobot status\t275.450671\t77.249248\t9.498900\t-0.540883\t-1.948178\t149.868265\t0.290000\t0.020000\n\t\n15:33:59.0\tlog_raw\tgps_raw\t\tsystem status\tnormal 2 28.000000 0 0\trobot status\t275.335658\t77.333857\t9.495700\t-0.446060\t-1.962362\t149.935090\t0.291000\t0.017000\n\t\n15:33:59.5\tlog_raw\tgps_raw\t#INSPVAXA,USB3,0,51.5,FINESTEERING,2107,282857.550,02008000,471d,15824;INS_ALIGNMENT_COMPLETE,INS_RTKFIXED,37.37082778753,126.72394219163,9.4923,22.3000,0.1642,-0.2009,-0.0151,-0.455107252,-1.810033780,299.964612436,0.4399,0.2940,0.5516,0.1134,0.0924,0.0772,0.0981,0.1030,4.8372,0f000001,0*479a7bb4\n\tsystem status\tnormal 2 28.000000 0 0\trobot status\t275.220636\t77.417330\t9.492300\t-0.455107\t-1.810034\t150.035388\t0.364000\t-0.116000\n\t\n15:34:00.0\tlog_raw\tgps_raw\t#INSPVAXA,USB3,0,49.5,FINESTEERING,2107,282858.050,02008000,471d,15824;INS_ALIGNMENT_COMPLETE,INS_RTKFIXED,37.37082854374,126.72394089011,9.4899,22.3000,0.1736,-0.2113,-0.0068,-0.453429457,-1.745153830,299.927988813,0.4398,0.2940,0.5516,0.1134,0.0924,0.0772,0.0981,0.1030,4.8386,0f000001,0*54a30be2\n\tsystem status\tnormal 2 28.000000 0 0\trobot status\t275.105349\t77.501261\t9.489900\t-0.453429\t-1.745154\t150.072011\t0.292000\t0.013000\n\t\n15:34:00.5\tlog_raw\tgps_raw\t\tsystem status\tnormal 2 28.000000 0 0\trobot status\t274.994222\t77.583267\t9.486700\t-0.354357\t-1.525474\t150.160218\t0.308000\t-0.011000\n\t\n15:34:01.0\tlog_raw\tgps_raw\t\tsystem status\tnormal 2 28.000000 0 0\trobot status\t274.879250\t77.667805\t9.482500\t-0.272264\t-1.557467\t150.234846\t0.351000\t-0.076000\n\t\n15:34:01.5\tlog_raw\tgps_raw\t#INSPVAXA,USB3,0,48.5,FINESTEERING,2107,282859.550,02008000,471d,15824;INS_ALIGNMENT_COMPLETE,INS_RTKFIXED,37.37083079066,126.72393699083,9.4791,22.3000,0.1717,-0.2000,-0.0121,-0.342154854,-1.629050926,299.761505256,0.4409,0.2941,0.5521,0.1136,0.0924,0.0772,0.0981,0.1030,4.8401,0f000001,0*7242c930\n\tsystem status\tnormal 2 28.000000 0 0\trobot status\t274.759957\t77.750646\t9.479100\t-0.342155\t-1.629051\t150.238495\t0.246000\t0.079000\n\t\n15:34:02.0\tlog_raw\tgps_raw\t#INSPVAXA,USB3,0,48.5,FINESTEERING,2107,282860.050,02008000,471d,15824;INS_ALIGNMENT_COMPLETE,INS_RTKFIXED,37.37083153175,126.72393569297,9.4766,22.3000,0.1682,-0.1931,-0.0033,-0.310568947,-1.805942662,299.681002094,0.4411,0.2941,0.5523,0.1135,0.0924,0.0772,0.0981,0.1030,4.8414,0f000001,0*16d456af\n\tsystem status\tnormal 2 28.000000 0 0\trobot status\t274.644995\t77.832900\t9.476600\t-0.310569\t-1.805943\t150.318998\t0.245000\t0.081000\n\t\n15:34:02.5\tlog_raw\tgps_raw\t#INSPVAXA,USB3,0,51.0,FINESTEERING,2107,282860.550,02000000,471d,15824;INS_ALIGNMENT_COMPLETE,INS_RTKFIXED,37.37083229529,126.72393437190,9.4736,22.3000,0.1681,-0.2003,0.0025,-0.225394302,-1.975265163,299.646950177,0.4411,0.2941,0.5523,0.1135,0.0924,0.0772,0.0981,0.1030,4.8414,0f000001,0*68c0c475\n\tsystem status\tnormal 2 28.000000 0 0\trobot status\t274.527977\t77.917645\t9.473600\t-0.225394\t-1.975265\t150.353050\t0.222000\t0.112000\n\t\n15:34:03.0\tlog_raw\tgps_raw\t\tsystem status\tnormal 2 28.000000 0 0\trobot status\t274.410875\t78.002778\t9.469900\t-0.208578\t-2.046636\t150.402526\t0.306000\t-0.003000\n\t\n15:34:03.5\tlog_raw\tgps_raw\t#INSPVAXA,USB3,0,49.5,FINESTEERING,2107,282861.550,02000000,471d,15824;INS_ALIGNMENT_COMPLETE,INS_RTKFIXED,37.37083383059,126.72393172727,9.4648,22.3000,0.1776,-0.2087,-0.0050,-0.195119204,-2.063452945,299.576804246,0.4408,0.2940,0.5521,0.1134,0.0924,0.0772,0.0981,0.1030,4.8426,0f000001,0*61c3be3c\n\tsystem status\tnormal 2 28.000000 0 0\trobot status\t274.293720\t78.088047\t9.464800\t-0.195119\t-2.063453\t150.423196\t0.302000\t0.006000\n\t\n15:34:04.0\tlog_raw\tgps_raw\t\tsystem status\tnormal 2 27.900000 0 0\trobot status\t274.181471\t78.171622\t9.459900\t-0.159106\t-1.955883\t150.500546\t0.265000\t0.052000\n\t\n15:34:04.5\tlog_raw\tgps_raw\t\tsystem status\tnormal 2 28.000000 0 0\trobot status\t274.062761\t78.257341\t9.456200\t-0.103884\t-1.989818\t150.576203\t0.229000\t0.094000\n\t\n15:34:05.0\tlog_raw\tgps_raw\t#INSPVAXA,USB3,0,43.5,FINESTEERING,2107,282863.050,02000000,471d,15824;INS_ALIGNMENT_COMPLETE,INS_RTKFIXED,37.37083613532,126.72392778169,9.4521,22.3000,0.1728,-0.2101,-0.0119,-0.074623458,-1.995146036,299.426549477,0.4414,0.2940,0.5522,0.1135,0.0924,0.0772,0.0981,0.1030,4.8451,0f000001,0*1428b524\n\tsystem status\tnormal 2 28.000000 0 0\trobot status\t273.944227\t78.343848\t9.452100\t-0.074623\t-1.995146\t150.573451\t0.296000\t0.005000\n\t\n15:34:05.5\tlog_raw\tgps_raw\t\tsystem status\tnormal 2 28.000000 0 0\trobot status\t273.825869\t78.428875\t9.447600\t-0.087258\t-2.081170\t150.622363\t0.249000\t0.074000\n\t\n15:34:06.0\tlog_raw\tgps_raw\t\tsystem status\tnormal 2 28.000000 0 0\trobot status\t273.710594\t78.513266\t9.443000\t-0.022384\t-2.036907\t150.642269\t0.347000\t-0.058000\n\t\n15:34:06.5\tlog_raw\tgps_raw\t\tsystem status\tnormal 2 28.000000 0 0\trobot status\t273.593222\t78.597278\t9.438600\t-0.063552\t-2.143674\t150.657093\t0.228000\t0.093000\n\t\n15:34:07.0\tlog_raw\tgps_raw\t\tsystem status\tnormal 2 28.000000 0 0\trobot status\t273.476258\t78.682434\t9.434800\t-0.087928\t-2.096760\t150.703907\t0.258000\t0.061000\n\t\n15:34:07.5\tlog_raw\tgps_raw\t\tsystem status\tnormal 2 28.000000 0 0\trobot status\t273.359688\t78.766352\t9.430800\t-0.078842\t-2.063511\t150.706443\t0.356000\t-0.080000\n\t\n15:34:08.0\tlog_raw\tgps_raw\t\tsystem status\tnormal 2 28.000000 0 0\trobot status\t273.243724\t78.849752\t9.427200\t-0.115635\t-2.127652\t150.767499\t0.273000\t0.043000\n\t\n15:34:08.5\tlog_raw\tgps_raw\t#INSPVAXA,USB3,0,51.5,FINESTEERING,2107,282866.550,02000000,471d,15824;INS_ALIGNMENT_COMPLETE,INS_RTKFIXED,37.37084144931,126.72391854288,9.4238,22.3000,0.1586,-0.1939,-0.0075,-0.000254507,-1.973115927,299.207530443,0.4415,0.2941,0.5523,0.1135,0.0924,0.0772,0.0981,0.1030,4.8486,0f000001,0*7419bcbe\n\tsystem status\tnormal 2 28.000000 0 0\trobot status\t273.125868\t78.933646\t9.423800\t-0.000255\t-1.973116\t150.792470\t0.239000\t0.069000\n\t\n15:34:09.0\tlog_raw\tgps_raw\t\tsystem status\tnormal 2 28.000000 0 0\trobot status\t273.009320\t79.017390\t9.421400\t0.006977\t-2.054136\t150.797381\t0.299000\t0.003000\n\t\n15:34:09.5\tlog_raw\tgps_raw\t\tsystem status\tnormal 2 28.000000 0 0\trobot status\t272.892949\t79.099487\t9.417600\t0.055261\t-2.091172\t150.855063\t0.278000\t0.030000\n\t\n15:34:10.0\tlog_raw\tgps_raw\t\tsystem status\tnormal 2 28.000000 0 0\trobot status\t272.776516\t79.181736\t9.413900\t-0.027341\t-1.963024\t150.887675\t0.311000\t-0.033000\n\t\n15:34:10.5\tlog_raw\tgps_raw\t\tsystem status\tnormal 2 28.000000 0 0\trobot status\t272.659895\t79.264794\t9.409700\t0.024933\t-1.856844\t150.874092\t0.375000\t-0.114000\n\t\n15:34:11.0\tlog_raw\tgps_raw\t\tsystem status\tnormal 2 28.000000 0 0\trobot status\t272.546705\t79.347001\t9.406500\t0.119134\t-1.737672\t150.963426\t0.268000\t0.054000\n\t\n15:34:11.5\tlog_raw\tgps_raw\t#INSPVAXA,USB3,0,49.0,FINESTEERING,2107,282869.550,02000000,471d,15824;INS_ALIGNMENT_COMPLETE,INS_RTKFIXED,37.37084591641,126.72391064457,9.4025,22.3000,0.1631,-0.2087,-0.0091,0.094919053,-1.740347092,299.016545288,0.4419,0.2942,0.5525,0.1136,0.0924,0.0772,0.0981,0.1030,4.8515,0f000001,0*b4375d21\n\tsystem status\tnormal 2 28.000000 0 0\trobot status\t272.426249\t79.429448\t9.402500\t0.094919\t-1.740347\t150.983455\t0.368000\t-0.110000\n\t\n15:34:12.0\tlog_raw\tgps_raw\t\tsystem status\tnormal 2 28.000000 0 0\trobot status\t272.307086\t79.510774\t9.398900\t-0.012880\t-1.693345\t150.931337\t0.245000\t0.067000\n\t\n15:34:12.5\tlog_raw\tgps_raw\t\tsystem status\tnormal 2 28.000000 0 0\trobot status\t272.184639\t79.593615\t9.396300\t-0.025859\t-1.845044\t150.927995\t0.292000\t0.005000\n\t\n15:34:13.0\tlog_raw\tgps_raw\t\tsystem status\tnormal 2 28.000000 0 0\trobot status\t272.065732\t79.676024\t9.394200\t0.017416\t-1.921323\t150.964022\t0.257000\t0.066000\n\t\n15:34:13.5\tlog_raw\tgps_raw\t\tsystem status\tnormal 2 28.000000 0 0\trobot status\t271.942617\t79.760236\t9.390200\t-0.005186\t-2.072102\t150.934635\t0.256000\t0.057000\n\t\n15:34:14.0\tlog_raw\tgps_raw\t\tsystem status\tnormal 2 28.000000 0 0\trobot status\t271.821229\t79.845630\t9.385900\t0.011116\t-2.081172\t150.833177\t0.287000\t0.013000\n\t\n15:34:14.5\tlog_raw\tgps_raw\t\tsystem status\tnormal 2 28.000000 0 0\trobot status\t271.701790\t79.929154\t9.383500\t-0.011080\t-2.049986\t150.826997\t0.296000\t0.015000\n\t\n15:34:15.0\tlog_raw\tgps_raw\t\tsystem status\tnormal 2 28.000000 0 0\trobot status\t271.582994\t80.011894\t9.381000\t-0.173677\t-1.974372\t150.809754\t0.360000\t-0.080000\n\t\n15:34:15.5\tlog_raw\tgps_raw\t\tsystem status\tnormal 2 28.000000 0 0\trobot status\t271.461318\t80.096882\t9.376900\t-0.188024\t-1.947057\t150.748449\t0.263000\t0.052000\n\t\n15:34:16.0\tlog_raw\tgps_raw\t\tsystem status\tnormal 2 28.000000 0 0\trobot status\t271.338992\t80.183786\t9.371900\t-0.213913\t-2.112951\t150.684285\t0.293000\t0.012000\n\t\n15:34:16.5\tlog_raw\tgps_raw\t\tsystem status\tnormal 2 28.000000 0 0\trobot status\t271.222547\t80.267561\t9.368400\t-0.121604\t-2.163348\t150.629617\t0.321000\t-0.019000\n\t\n15:34:17.0\tlog_raw\tgps_raw\t\tsystem status\tnormal 2 28.000000 0 0\trobot status\t271.098325\t80.356093\t9.364500\t-0.190895\t-2.343957\t150.470985\t0.337000\t-0.069000\n\t\n15:34:17.5\tlog_raw\tgps_raw\t\tsystem status\tnormal 2 28.000000 0 0\trobot status\t270.977083\t80.441548\t9.360600\t-0.234319\t-2.235845\t150.362889\t0.327000\t-0.031000\n\t\n15:34:18.1\tlog_raw\tgps_raw\t\tsystem status\tnormal 2 28.000000 0 0\trobot status\t270.861185\t80.525110\t9.356200\t-0.307520\t-2.205290\t150.295582\t0.371000\t-0.104000\n\t\n15:34:18.6\tlog_raw\tgps_raw\t\tsystem status\tnormal 2 28.000000 0 0\trobot status\t270.743059\t80.610044\t9.351700\t-0.334966\t-2.094021\t150.291197\t0.257000\t0.050000\n\t\n15:34:19.0\tlog_raw\tgps_raw\t\tsystem status\tnormal 2 28.000000 0 0\trobot status\t270.622972\t80.698690\t9.346300\t-0.180992\t-1.994468\t150.258343\t0.241000\t0.075000\n\t\n15:34:19.5\tlog_raw\tgps_raw\t\tsystem status\tnormal 2 28.000000 0 0\trobot status\t270.505216\t80.782206\t9.342500\t-0.209157\t-2.014220\t150.240852\t0.387000\t-0.126000\n\t\n15:34:20.1\tlog_raw\tgps_raw\t\tsystem status\tnormal 2 28.000000 0 0\trobot status\t270.387124\t80.867498\t9.338400\t-0.169498\t-1.949403\t150.266477\t0.300000\t0.013000\n\t\n15:34:20.6\tlog_raw\tgps_raw\t\tsystem status\tnormal 2 28.000000 0 0\trobot status\t270.268666\t80.951884\t9.332500\t-0.114786\t-2.010062\t150.241401\t0.247000\t0.063000\n\t\n15:34:21.1\tlog_raw\tgps_raw\t\tsystem status\tnormal 2 28.000000 0 0\trobot status\t270.149471\t81.037067\t9.326800\t-0.108903\t-2.133388\t150.264628\t0.240000\t0.074000\n\t\n15:34:21.6\tlog_raw\tgps_raw\t\tsystem status\tnormal 2 28.000000 0 0\trobot status\t270.029764\t81.120186\t9.320600\t-0.302248\t-2.134462\t150.297957\t0.236000\t0.091000\n\t\n15:34:22.1\tlog_raw\tgps_raw\t\tsystem status\tnormal 2 28.000000 0 0\trobot status\t269.910504\t81.204121\t9.315700\t-0.399493\t-2.331646\t150.398580\t0.257000\t0.079000\n\t\n15:34:22.6\tlog_raw\tgps_raw\t\tsystem status\tnormal 2 27.900000 0 0\trobot status\t269.794045\t81.285974\t9.310000\t-0.375228\t-2.245719\t150.470655\t0.402000\t-0.154000\n\t\n15:34:23.1\tlog_raw\tgps_raw\t\tsystem status\tnormal 2 28.000000 0 0\trobot status\t269.676126\t81.370009\t9.303800\t-0.184391\t-2.150518\t150.499144\t0.271000\t0.049000\n\t\n15:34:23.6\tlog_raw\tgps_raw\t\tsystem status\tnormal 2 28.000000 0 0\trobot status\t269.554765\t81.451555\t9.296800\t-0.326012\t-2.137247\t150.562283\t0.288000\t0.028000\n\t\n15:34:24.1\tlog_raw\tgps_raw\t\tsystem status\tnormal 2 28.000000 0 0\trobot status
